vi "DFD Elliptic Order Estimation.vi"(6 "fs [Hz]":dbl=1.0 format="%.2f", 7 "filter type":T4(ring), 8 "error in (no error)":errorcluster, 10 "ripple specs":T1={"passband"=0.1, "stopband"=60.0, "dB/linear? (T: dB)"=TRUE}, 11 "freq specs [Hz]":T2={"fpass 1"=0.2, "fstop 1"=0.3, "fpass 2 "=0.0, "fstop 2"=0.0}) -> (0 "error out":errorcluster, 1 "low cutoff freq [Hz]":dbl, 2 "high cutoff freq [Hz]":dbl, 3 "estimated order":i32, 4 "ripples [dB]":T3={"passband ripple"=1.0, "stopband atten"=60.0} {"stopband atten" format="%.2f"; "passband ripple" format="%.2f"})   [LabVIEW 2017, in "NI_DigFilterLicensed.lvlib"]
doc: "Estimates the Elliptic filter order."
uses:
  <vilib>/addons/Digital Filter Design/NI_DigFilterLicensed.lvlib
  <vilib>/addons/Digital Filter Design/_Objects.llb/DFD Filter Frequence Specification (Design).ctl
  <vilib>/addons/Digital Filter Design/_Objects.llb/DFD Filter Ripple Specification (Design).ctl
  <vilib>/addons/Digital Filter Design/NI_DigFilter_Design.lvlib
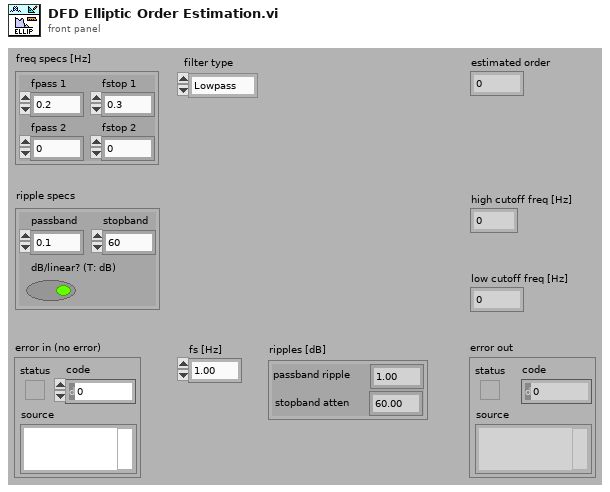
[diagram p1: front panel]
types:
  T1 = typedef "NI_DigFilterLicensed.lvlib/DFD Filter Ripple Specification (Design).ctl" = cluster{"passband":dbl, "stopband":dbl, "dB/linear? (T: dB)":bool}
  T2 = typedef "NI_DigFilterLicensed.lvlib/DFD Filter Frequence Specification (Design).ctl" = cluster{"fpass 1":dbl, "fstop 1":dbl, "fpass 2 ":dbl, "fstop 2":dbl}
  T3 = cluster{"passband ripple":dbl, "stopband atten":dbl}
  T4 = enum16{"Lowpass", "Highpass", "Bandpass", "Bandstop"}
  T5 = enum16{"Butterworth", "Chebyshev", "Inverse Chebyshev", "Elliptic", "Bessel"}
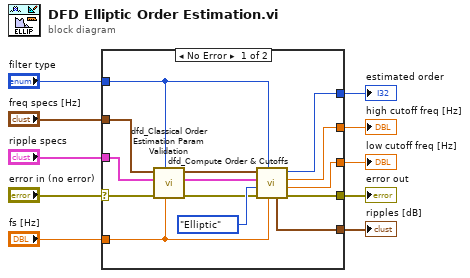
[diagram p0: block diagram]
diagram:
  n1 = case shown="No Error" "error in (no error)" {
    selector: "error in (no error)" -> [w11 w25]
    tunnel: "fs [Hz]" -> [w24 _]
    tunnel: "filter type" -> [w23 _]
    tunnel: [w21 w25] -> w8
    tunnel: [w17 _] -> w7
    tunnel: "ripple specs" -> [w16 _]
    tunnel: "freq specs [Hz]" -> [w15 _]
    tunnel: [w14 _] -> w4
    tunnel: [w13 _] -> w3
    tunnel: [w12 _] -> w2
    frame No Error {
      n2 = call <vilib>:"dfd_Classical Order Estimation Param Validation.vi"("fs [Hz]"=w24, "filter type"=w23, "error in (no error)"=w11, "ripple specs"=w16, "freq specs [Hz]"=w15) -> ("error out"=w20:errorcluster, "dup ripple specs"=w18:T1, "dup freq specs [Hz]"=w19:T2)  [unwired: 1 in, 3 out]
      n3 = call <vilib>:"dfd_Compute Order & Cutoffs.vi"("fs [Hz]"=w24, "filter type"=w23, "error in (no error)"=w20, "design method"=T5."Elliptic", "ripple specs"=w18, "freq specs [Hz]"=w19) -> ("error out"=w21:errorcluster, "low cutoff freq: fl"=w12:dbl, "high cutoff freq: fh"=w13:dbl, "N"=w14:i32, "ripples [dB]"=w17:T3)  [unwired: 1 out]
    }
    frame Error {
    }
  }
  "estimated order" <- w4
  "error out" <- w8
  "ripples [dB]" <- w7
  "high cutoff freq [Hz]" <- w3
  "low cutoff freq [Hz]" <- w2
